vi "Execute (no results).vi"(8 "error in (no error)":errorcluster, 10 "SQL":string, 11 "PQ Connection in":refnum<class "PQ Connection.lvclass">) -> (0 "error out":errorcluster, 3 "PQ Connection out":refnum<class "PQ Connection.lvclass">)   [LabVIEW 2016, in "PQ Connection.lvclass"]
uses:
  PQ Connection.lvclass
  Result/PQ Result.lvclass
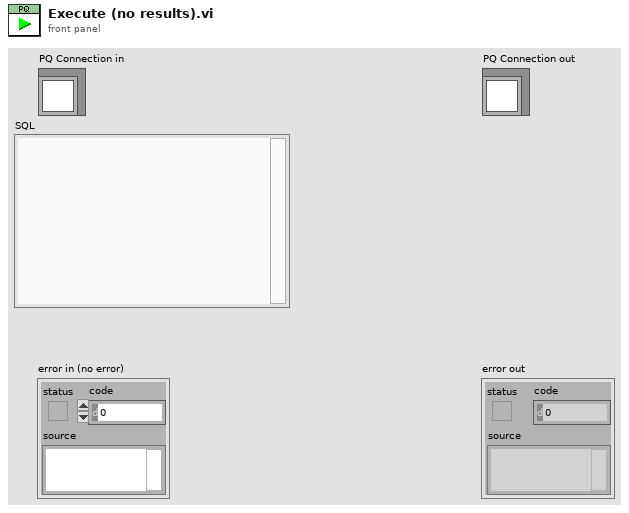
[diagram p1: front panel]
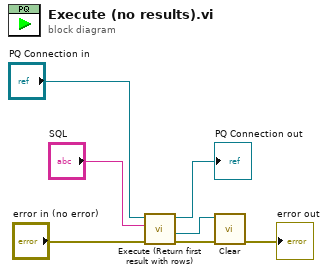
[diagram p0: block diagram]
diagram:
  n1 = call "Execute (Return first result with rows).vi"("error in (no error)"="error in (no error)", "SQL"="SQL", "PQ Connection in"="PQ Connection in") -> ("error out"=w1:errorcluster, "First Result with Rows returned"=w2:refnum<class "PQ Result.lvclass">, "PQ Connection out"=→"PQ Connection out":refnum<class "PQ Connection.lvclass">)  [unwired: 5 in, 1 out]
  n2 = call "Clear.vi"("error in (no error)"=w1, "PQ Result  in"=w2) -> ("error out"=→"error out":errorcluster)  [unwired: 9 in]
